vi "AvailableRecords.vi"(10 "5782 records":u16[](array[numeric]), 11 "5160 records":i32[](array[numeric])) -> (1 "last record size 5782":u32, 2 "#elements 5782":u32, 3 "record available":bool, 5 "last record size 5160":u32, 7 "#elements 5160":u32)   [LabVIEW 2013]
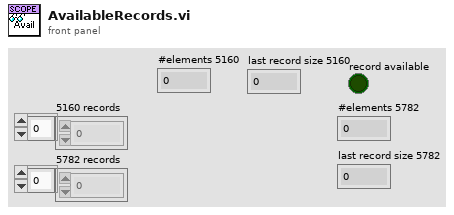
[diagram p1: front panel]
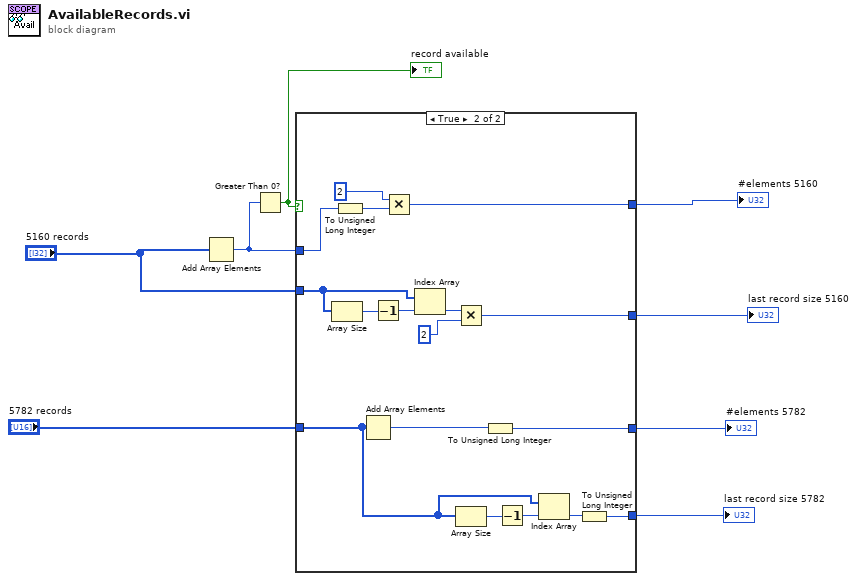
[diagram p0: block diagram]
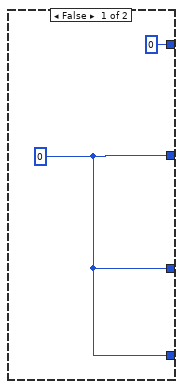
[diagram p2: hidden frame]
diagram:
  n1 = Add Array Elements(numeric array="5160 records") -> (sum=w8:i32)
  n2 = Greater Than 0?(x=w8) -> (x > 0?=w7:bool)
  "record available" <- w7
  n3 = case shown="True" w7 {
    tunnel: w8 -> [_ w24]
    tunnel: "5160 records" -> [_ w27]
    tunnel: [w9 w19] -> w6
    tunnel: [u32 0 w18] -> w5
    tunnel: "5782 records" -> [_ w14]
    tunnel: [w9 w13] -> w4
    tunnel: [w9 w11] -> w3
    frame False {
      w9 = u32 0
    }
    frame True {
      n4 = Array Size(array=w27) -> (size(s)=w26:i32)
      n5 = To Unsigned Long Integer(number=w24) -> (unsigned 32bit integer=w23:u32)
      n6 = Add Array Elements(numeric array=w14) -> (sum=w17:u16)
      n7 = Decrement(x=w26) -> (x-1=w25:i32)
      n8 = Multiply(x=u32 2, y=w23) -> (x*y=w18:u32)
      n9 = Index Array(array=w27, index=w25) -> (element=w21:i32)
      n10 = Multiply(x=w21, y=u32 2 ("x")) -> (x*y=w19:u32)
      n11 = Array Size(array=w14) -> (size(s)=w16:i32)
      n12 = To Unsigned Long Integer(number=w17) -> (unsigned 32bit integer=w13:u32)
      n13 = Decrement(x=w16) -> (x-1=w15:i32)
      n14 = Index Array(array=w14, index=w15) -> (element=w12:u16)
      n15 = To Unsigned Long Integer(number=w12) -> (unsigned 32bit integer=w11:u32)
    }
  }
  "last record size 5160" <- w6
  "#elements 5160" <- w5
  "last record size 5782" <- w3
  "#elements 5782" <- w4
